vi "Compteur.vi"(8 "error in (no error)":errorcluster, 11 "Caller in":refnum<class "Caller.lvclass">) -> (0 "error out":errorcluster, 3 "Caller out":refnum<class "Caller.lvclass">)   [LabVIEW 2020, in "Caller.lvlib" / "Caller.lvclass"]
uses:
  Caller.lvclass
  Caller.lvclass/Caller.ctl
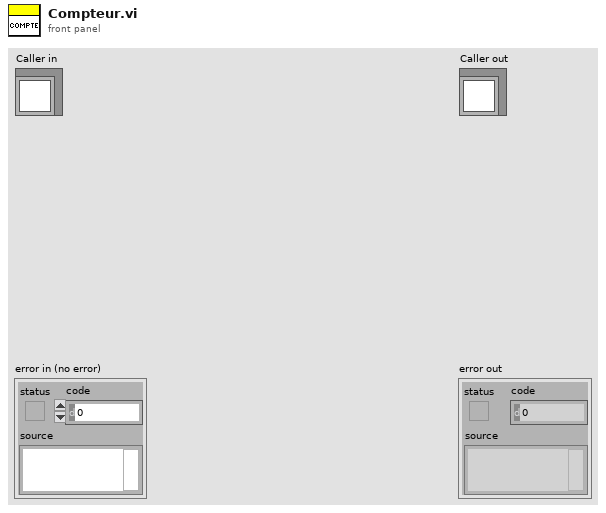
[diagram p1: front panel]
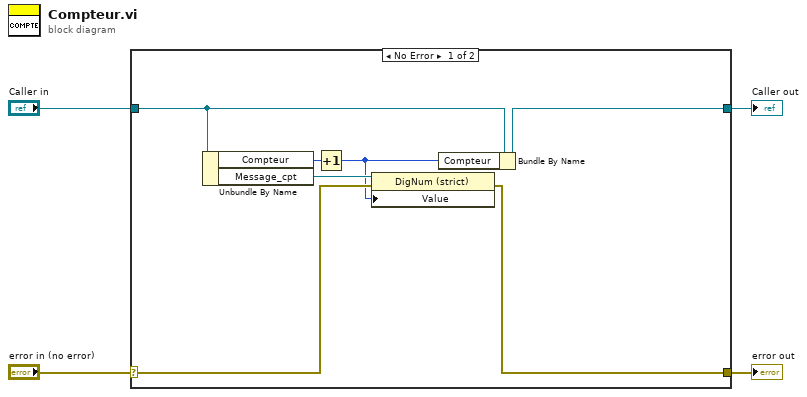
[diagram p0: block diagram]
diagram:
  n1 = case shown="No Error" "error in (no error)" {
    selector: "error in (no error)" -> [w7 w13]
    tunnel: [w6 w13] -> w3
    tunnel: [w9 w12] -> w1
    tunnel: "Caller in" -> [w11 w12]
    frame No Error {
      n2 = Unbundle By Name(w11) -> ("Compteur"=w10:u8, "Message_cpt"=w8:refnum<vi>)
      n3 = Increment(x=w10) -> (x+1=w5:u8)
      n4 = property class="DigNum (strict)"(reference=w8, error in=w7, "Value"=w5) -> (error out=w6:errorcluster)  [unwired: 1 out]
      n5 = Bundle By Name(cluster=w11, "Compteur"=w5) -> (w9:refnum<class "Caller.lvclass">)
    }
    frame Error {
    }
  }
  "error out" <- w3
  "Caller out" <- w1
